vi "Stop Sequence.vi"(8 "error in (no error)":errorcluster, 11 "Iteration Actions in":refnum<class "Iteration Actions.lvclass">) -> (0 "error out":errorcluster, 3 "Iteration Actions out":refnum<class "Iteration Actions.lvclass">)   [LabVIEW 2020, in "VolatusSeq.lvlib" / "Iteration Actions.lvclass"]
uses:
  Iteration Actions.lvclass
  Iteration Actions.lvclass/Iteration Actions.ctl
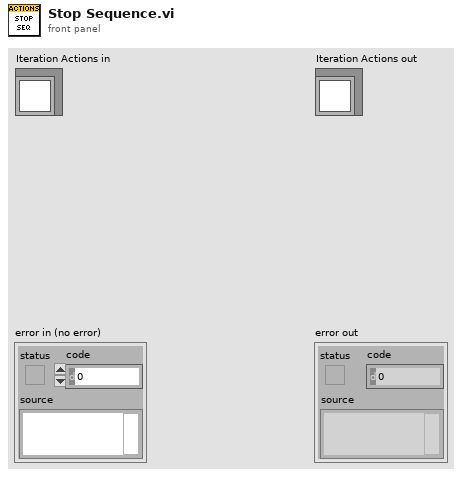
[diagram p1: front panel]
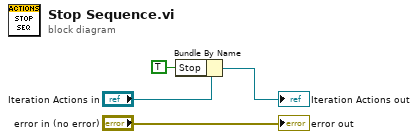
[diagram p0: block diagram]
diagram:
  n1 = Bundle By Name(cluster="Iteration Actions in", "Stop"=TRUE) -> (→"Iteration Actions out":refnum<class "Iteration Actions.lvclass">)
  "error out" <- "error in (no error)"
